vi "SetAttenuation.vi"(2 "error in (no error)":errorcluster, 3 "Attenuation (dB)":i32 min=0 max=120 step=1 format="%_3g") -> (0 "error out":errorcluster)   [LabVIEW 2009]
doc: "Parses the requested attenuation then builds the SCPI command list"
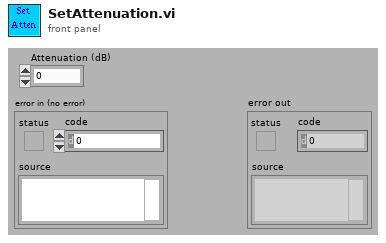
[diagram p1: front panel]
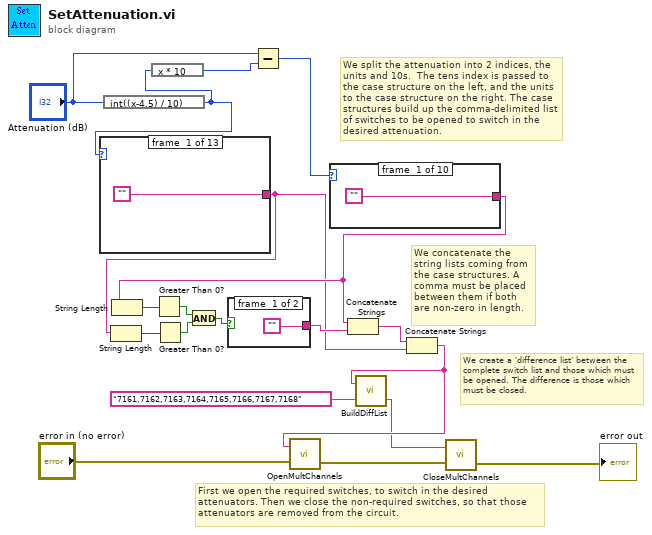
[diagram p0: block diagram]
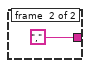
[diagram p2: hidden frame]
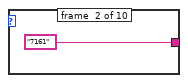
[diagram p3: hidden frame]
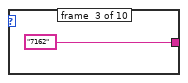
[diagram p4: hidden frame]
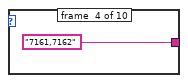
[diagram p5: hidden frame]
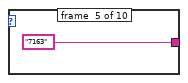
[diagram p6: hidden frame]
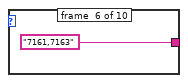
[diagram p7: hidden frame]
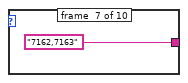
[diagram p8: hidden frame]
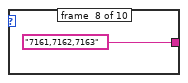
[diagram p9: hidden frame]
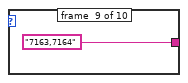
[diagram p10: hidden frame]
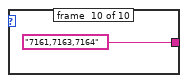
[diagram p11: hidden frame]
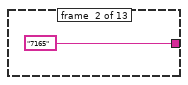
[diagram p12: hidden frame]
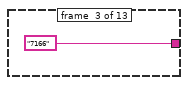
[diagram p13: hidden frame]
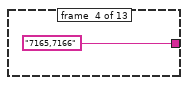
[diagram p14: hidden frame]
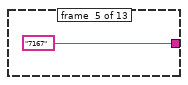
[diagram p15: hidden frame]
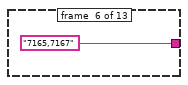
[diagram p16: hidden frame]
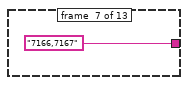
[diagram p17: hidden frame]
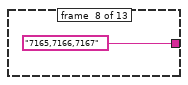
[diagram p18: hidden frame]
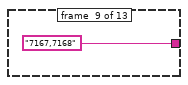
[diagram p19: hidden frame]
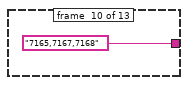
[diagram p20: hidden frame]
diagram:
  # "First we open the required switches, to switch in the desired attenuators. Then we close the non-required switches, so that those attenuators are removed from the circuit."
  # "We create a 'difference list' between the complete switch list and those which must be opened. The difference is those which must be closed."
  # "We concatenate the string lists coming from the case structures. A comma must be placed between them if both are non-zero in length."
  # "We split the attenuation into 2 indices, the units and 10s.  The tens index is passed to the case structure on the left, and the units to the case structure on the right. The case structures build up the comma-delimited list of switches to be opened to switch in the desired attenuation."
  n1 = expression code="int((x-4.5) / 10)"("Attenuation (dB)") -> (w18:i32)
  n2 = case shown="12" w18 {
    tunnel: ["" "7165" "7166" "7165,7166" "7167" "7165,7167" "7166,7167" "7165,7166,7167" "7167,7168" "7165,7167,7168" "7166,7167,7168" "7165,7166,7167,7168" w32] -> w9
    frame #0 {
    }
    frame #1 {
    }
    frame #2 {
    }
    frame #3 {
    }
    frame #4 {
    }
    frame #5 {
    }
    frame #6 {
    }
    frame #7 {
    }
    frame #8 {
    }
    frame #9 {
    }
    frame #10 {
    }
    frame #11 {
    }
    frame #12 {
      n3 = Concatenate Strings("7161,7162,7163,7164,", "7165,7166,7167,7168") -> (w32:string)
    }
  }
  n4 = String Length(string=w9) -> (length=w15:i32)
  n5 = expression code="x * 10"(w18) -> (w17:i32)
  n6 = Greater Than 0?(x=w15) -> (x > 0?=w6:bool)
  n7 = Subtract(x="Attenuation (dB)", y=w17) -> (x-y=w16:i32)
  n8 = case shown="0, Default" w16 {
    tunnel: ["" "7161" "7162" "7161,7162" "7163" "7161,7163" "7162,7163" "7161,7162,7163" "7163,7164" "7161,7163,7164"] -> w11
    frame #0 {
    }
    frame #1 {
    }
    frame #2 {
    }
    frame #3 {
    }
    frame #4 {
    }
    frame #5 {
    }
    frame #6 {
    }
    frame #7 {
    }
    frame #8 {
    }
    frame #9 {
    }
  }
  n9 = String Length(string=w11) -> (length=w12:i32)
  n10 = Greater Than 0?(x=w12) -> (x > 0?=w7:bool)
  n11 = And(x=w7, y=w6) -> (x .and. y?=w10:bool)
  n12 = case shown="False" w10 {
    tunnel: ["" ","] -> w14
    frame #0 {
    }
    frame #1 {
    }
  }
  n13 = Concatenate Strings(w11, w14) -> (w13:string)
  n14 = Concatenate Strings(w13, w9) -> (w2:string)
  n15 = call "OpenMultChannels.vi"("error in (no error)"="error in (no error)", "Channels to be opened"=w2) -> ("error out"=w4:errorcluster)  [unwired: 1 in]
  n16 = call "BuildDiffList.vi"("Reference list"="7161,7162,7163,7164,7165,7166,7167,7168", "Input list"=w2) -> ("Difference list"=w1:string)  [unwired: 1 in]
  n17 = call "CloseMultChannels.vi"("error in (no error)"=w4, "Channels to be closed"=w1) -> ("error out"=→"error out":errorcluster)  [unwired: 1 in]
